vi "Yaw Pitch Roll from NI Apriltag code.vi"(6 "Tag ID":i32, 9 "Robot Calibration Cluster":T1={"Camera FOV Vert View Angle (deg)"=53.5, "Camera FOV Hor View Angle (deg)"=92.0, "Distance Correction Factor"=3.952} {"Distance Correction Factor" format="%#_13g"; "Camera FOV Hor View Angle (deg)" format="%#_13g"; "Camera FOV Vert View Angle (deg)" format="%#_13g"}, 10 "Homography H":dbl[](array[numeric]), 11 "Picture Cluster":cluster{"X Resolution":i32, "Y Resolution":i32}) -> (0 "Roll":dbl, 1 "Pitch":dbl, 2 "Yaw":dbl, 3 "Tag Center Distance (in)":dbl, 4 "Drive Distance (in)":dbl, 5 "Distance (tag-size units)":dbl)   [LabVIEW 2025]
uses:
  Camera Info.ctl
  Calculate Focal Lengths in Pixels.vi
panel:
  out "Homography H Matrix":dbl[][](array[numeric])
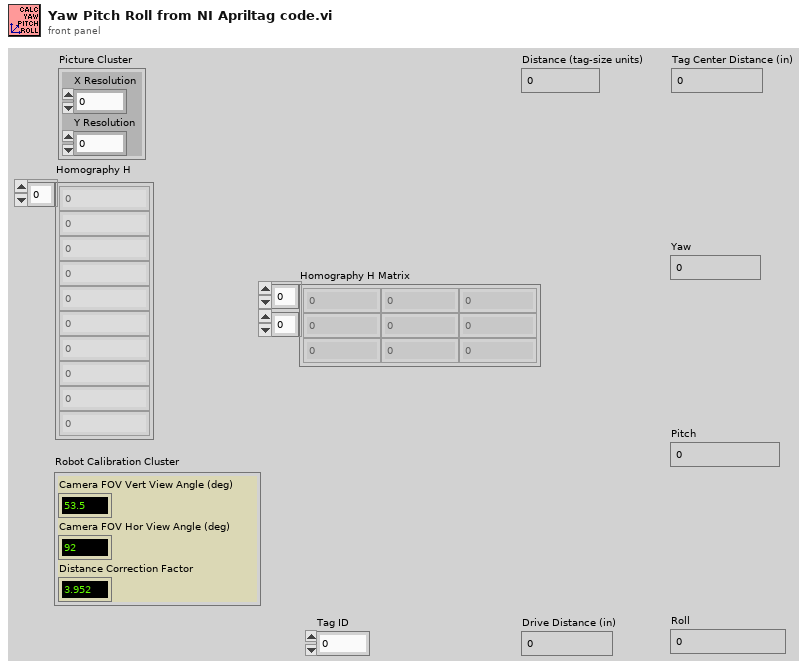
[diagram p1: front panel]
types:
  T1 = typedef "Camera Info.ctl" = cluster{"Camera FOV Vert View Angle (deg)":dbl, "Camera FOV Hor View Angle (deg)":dbl, "Distance Correction Factor":dbl}
  T2 = typedef "NI_Matrix.lvlib/RealMatrix.ctl" = dbl[][]
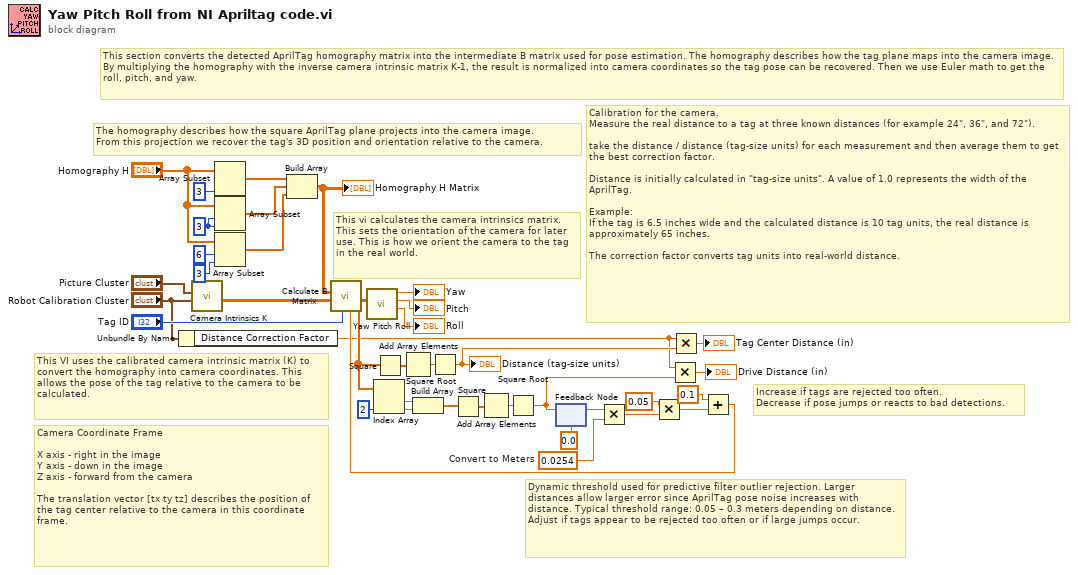
[diagram p0: block diagram]
diagram:
  w4 = 0.0254  # Convert to Meters
  w32 = 3 ("length")
  # "Increase if tags are rejected too often.\nDecrease if pose jumps or reacts to bad detections."
  # "Dynamic threshold used for predictive filter outlier rejection. Larger distances allow larger error since AprilTag pose noise increases with distance. Typical threshold range: 0.05 – 0.3 meters depending on distance. Adjust if tags appear to be rejected too often or if large jumps occur."
  # "Camera Coordinate Frame\n\nX axis - right in the image\nY axis - down in the image\nZ axis - forward from the camera\n\nThe translation vector [tx ty tz] describes the position of the tag center relative to the camera in this coordinate frame."
  # "This vi calculates the camera intrinsics matrix. This sets the orientation of the camera for later use. This is how we orient the camera to the tag in the real world."
  # "This VI uses the calibrated camera intrinsic matrix (K) to convert the homography into camera coordinates. This allows the pose of the tag relative to the camera to be calculated."
  # "The homography describes how the square AprilTag plane projects into the camera image.\nFrom this projection we recover the tag's 3D position and orientation relative to the camera."
  # "This section converts the detected AprilTag homography matrix into the intermediate B matrix used for pose estimation. The homography describes how the tag plane maps into the camera image. By multiplying the homography with the inverse camera intrinsic matrix K-1, the result is normalized into camera coordinates so the tag pose can be recovered. Then we use Euler math to get the roll, pitch, and yaw."
  # "Calibration for the camera. \nMeasure the real distance to a tag at three known distances (for example 24\", 36\", and 72\").\n\ntake the distance / distance (tag-size units) for each measurement and then average them to get the best correction factor.\n\nDistance is initially calculated in \"tag-size units\". A value of 1.0 represents the width of the AprilTag.\n\nExample:\nIf the tag is 6.5 inches wide and the calculated distance is 10 tag units, the real distance is approximately 65 inches.\n\nThe correction factor converts tag units into real-world distance."
  n1 = Unbundle By Name("Robot Calibration Cluster") -> ("Distance Correction Factor"=w2:dbl)
  n2 = call "Camera Intrinsics K.vi"("Robot Calibration Cluster"="Robot Calibration Cluster", "Picture Cluster"="Picture Cluster") -> ("Camera intrinsic matrix (K^-1)"=w39:dbl[][])  [unwired: 8 in, 1 out]
  n3 = Array Subset(array="Homography H", length=3) -> (w30:dbl[])  [unwired: 1 in]
  n4 = Array Subset(array="Homography H", index=w32, length=w32) -> (w25:dbl[])
  n5 = Array Subset(array="Homography H", index=6, length=3) -> (w29:dbl[])
  n6 = Build Array(w30, w25, w29) -> (w27:dbl[][])
  "Homography H Matrix" <- w27
  n7 = feedback #1(0.0) -> (w7:dbl)
  n8 = Multiply(x=w7, y=w4) -> (x*y=w5:dbl)
  n9 = Multiply(x=0.05, y=w5) -> (x*y=w8:dbl)
  n10 = Add(x=0.1, y=w8) -> (x+y=w6:dbl)
  n11 = call "Calculate B Matrix.vi"("threshold"=w6, "Tag ID"="Tag ID", "Camera intrinsic matrix (K^-1)"=w39, "Homography H"=w27) -> ("t (Translation Vector)"=w17:dbl[], "R Rotation Matrix (final)"=w38:T2)  [unwired: 5 in, 1 out]
  n12 = call "Yaw Pitch Roll.vi"("R Rotation Matrix"=w38) -> ("Roll"=→"Roll":dbl, "Pitch"=→"Pitch":dbl, "Yaw"=→"Yaw":dbl)  [unwired: 8 in]
  n13 = Index Array(array=w17, index #2=2 ("index")) -> (element #1=w14:dbl, element #2=w15:dbl)  [unwired: 1 in]
  n14 = Square(x=w17) -> (x^2=w23:dbl[])
  n15 = Add Array Elements(numeric array=w23) -> (sum=w22:dbl)
  n16 = Build Array(w14, w15) -> (w13:dbl[])
  n17 = Square Root(x=w22) -> (sqrt(x)=w21:dbl)
  "Distance (tag-size units)" <- w21
  n18 = Square(x=w13) -> (x^2=w19:dbl[])
  n19 = Add Array Elements(numeric array=w19) -> (sum=w20:dbl)
  n20 = Square Root(x=w20) -> (sqrt(x)=w11:dbl)
  n21 = feedback-in #1(w11) -> ()
  n22 = Multiply(x=w2, y=w11) -> (x*y=→"Drive Distance (in)":dbl)
  n23 = Multiply(x=w2, y=w21) -> (x*y=→"Tag Center Distance (in)":dbl)
